vi "Restart Unit.vi"(8 "error in (no error)":errorcluster, 10 "New IP (empty = original)":string, 11 "ENET in":refnum<class "ENET_BS1201.lvclass">) -> (0 "error out":errorcluster, 3 "ENET out":refnum<class "ENET_BS1201.lvclass">)   [LabVIEW 2021]
uses:
  ENET_BS1201.lvclass
  C:/Users/Public/Documents/Projects/7100-00109 SW BS1201 LV Driver/trunk/source/ENET_BS120x/ENET_BS120x.lvclass
  C:/Users/Public/Documents/Projects/7100-00109 SW BS1201 LV Driver/trunk/source/BS120x.lvclass
  C:/Users/Public/Documents/Projects/7100-00109 SW BS1201 LV Driver/trunk/source/ENET_BS1201/ENET_BS1201.lvclass
panel:
  out "Num Tries":i32
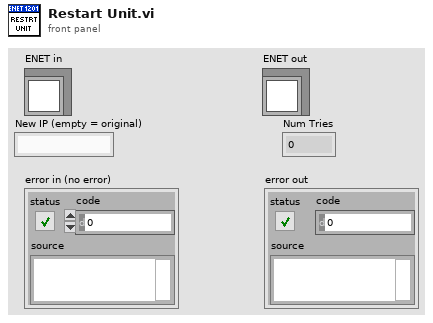
[diagram p1: front panel]
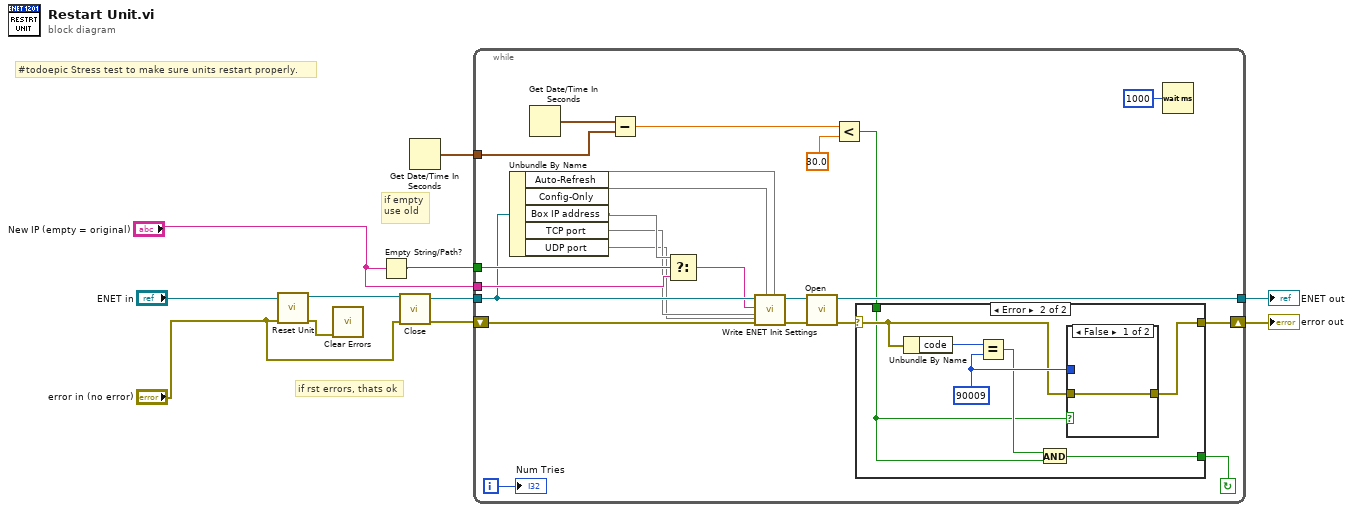
[diagram p0: block diagram]
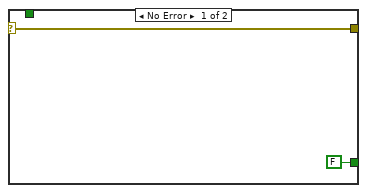
[diagram p2: hidden frame]
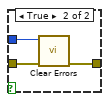
[diagram p3: hidden frame]
diagram:
  # "if rst errors, thats ok"
  # "if empty\nuse old"
  # "#todoepic Stress test to make sure units restart properly."
  n1 = call-dynamic "Reset Unit.vi"("error in (no error)"="error in (no error)", "Ethernet in"="ENET in") -> ("error out"=w2:errorcluster, "Ethernet out"=w7:refnum<class "ENET_BS1201.lvclass">)  [unwired: 8 in]
  n2 = call <vilib>:"Clear Errors.vi"("error in (no error)"=w2) -> ()  [unwired: 5 in, 2 out]
  n3 = Empty String/Path?(string/path="New IP (empty = original)") -> (empty?=w4:bool)
  n4 = call-dynamic "Close.vi"("error in (no error)"="error in (no error)", "ENET in"=w7) -> ("error out"=w5:errorcluster, "ENET out"=w6:refnum<class "ENET_BS1201.lvclass">)  [unwired: 8 in]
  n5 = Get Date/Time In Seconds() -> (seconds since 1Jan1904=w9:timestamp)
  n6 = while {
    tunnel: [w34] -> w10
    tunnel: w6 -> [w18]
    shift-right: [w33] -> w11
    shift-left: w5 -> [w17]
    tunnel: w9 -> [w31]
    tunnel: w4 -> [w23]
    tunnel: "New IP (empty = original)" -> [w21]
    i -> [w24]
    stop <- w26 continue-if-true
    n7 = Unbundle By Name(w18) -> ("Auto-Refresh"=w16, "Config-Only"=w15, "Box IP address"=w22, "TCP port"=w13, "UDP port"=w12)
    n8 = Get Date/Time In Seconds() -> (seconds since 1Jan1904=w32:timestamp)
    n9 = Subtract(x=w32, y=w31) -> (x-y=w30:dbl)
    n10 = Select(t=w22, s=w23, f=w21) -> (s? t:f=w14:string)
    n11 = call-dynamic "Write ENET Init Settings.vi"("Auto-Refresh (T)"=w16, "UDP port"=w12, "Connect for Config Only? (F)"=w15, "error in (no error)"=w17, "TCP port"=w13, "Box IP address"=w14, "Ethernet_BS1201 in"=w18) -> ("error out"=w19:errorcluster, "Ethernet_BS1201 out"=w20:refnum<class "ENET_BS1201.lvclass">)  [unwired: 3 in]
    n12 = call-dynamic "Open.vi"("error in (no error)"=w19, "ENET In"=w20) -> ("error out"=w28:errorcluster, "ENET out"=w34:refnum<class "ENET_BS1201.lvclass">)  [unwired: 8 in]
    n13 = Less?(x=w30, y=30.0) -> (x < y?=w27:bool)
    n14 = case shown="Error" w28 {
      selector: w28 -> [w36 w40]
      tunnel: [w36 w42] -> w33
      tunnel: w27 -> [_ w37]
      tunnel: [FALSE w38] -> w26
      frame No Error {
      }
      frame Error {
        w41 = 90009 ("y")
        n15 = Unbundle By Name(w40) -> ("code"=w43:i32)
        n16 = Equal?(x=w43, y=w41) -> (x = y?=w39:bool)
        n17 = And(x=w39, y=w37) -> (x .and. y?=w38:bool)
        n18 = case shown="False" w37 {
          tunnel: [w44 w47] -> w42
          tunnel: w41 -> [_ w46]
          tunnel: w40 -> [w44 w45]
          frame False {
          }
          frame True {
            n19 = call <vilib>:"Clear Errors.vi"("error in (no error)"=w45, "specific error code to clear (0: all)"=w46) -> ("error out"=w47:errorcluster)  [unwired: 4 in, 1 out]
          }
        }
      }
    }
    n20 = Wait (ms)(milliseconds to wait=u32 1000) -> ()  [unwired: 1 out]
    "Num Tries" <- w24
  }
  "error out" <- w11
  "ENET out" <- w10
